vi "Test Error.vi"(11 "Parametrized Test Case Test Double In":refnum<class "Parametrized Test Case Test Double.lvclass">) -> (0 "error out":errorcluster, 3 "Parametrized Test Case Test Double Out":refnum<class "Parametrized Test Case Test Double.lvclass">)   [LabVIEW 2020, in "Parametrized Test Case Test Double.lvclass"]
uses:
  Parametrized Test Case Test Double.lvclass
  C:/Program Files (x86)/National Instruments/LabVIEW 2020/vi.lib/Astemes/LUnit/Test Case.lvclass
  <vilib>/Astemes/LUnit/Test Case.lvclass/Test Case.ctl
  <vilib>/Astemes/LUnit/Append Fail Result.vi
  <vilib>/Astemes/LUnit/Run In UI.vi
  <vilib>/Utility/error.llb/Clear Errors.vi
  <vilib>/Astemes/LUnit/Test Case.lvclass
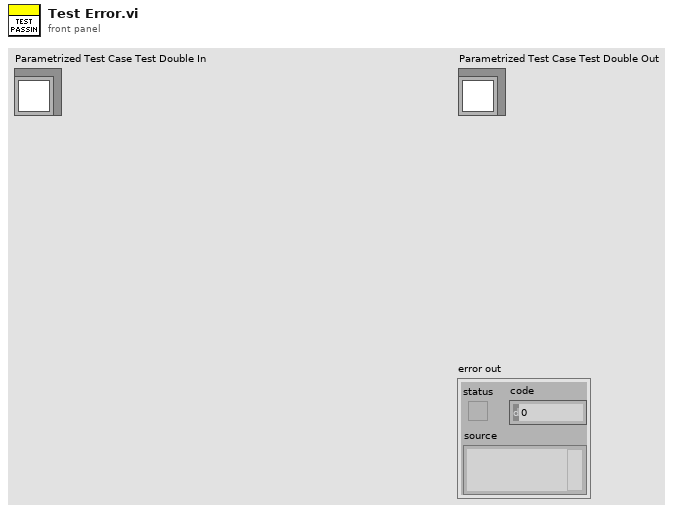
[diagram p1: front panel]
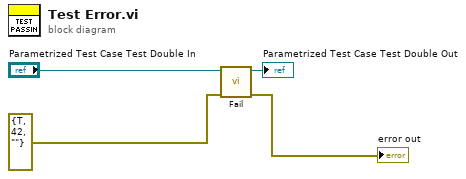
[diagram p0: block diagram]
diagram:
  n1 = call <vilib>:"Fail.vi"("error in (no error)"=errorcluster {"status"=TRUE, "code"=42, "source"=""} ("error out"), "LUnit Test Case In"="Parametrized Test Case Test Double In") -> ("error out"=→"error out":errorcluster, "LUnit Test Case Out"=→"Parametrized Test Case Test Double Out":refnum<class "Parametrized Test Case Test Double.lvclass">)  [unwired: 8 in]
